vi "ClientNTTestUpdate.vi"(8 "NT Connection":bool, 9 "CreateTestNew":bool, 10 "Flush0":bool, 11 "TestConfig":T1) -> (0 "Value3":dbl, 1 "Value2":dbl, 2 "Value1":dbl, 3 "Value0":dbl, 4 "Good2":bool, 5 "Good1":bool, 6 "Good3":bool, 7 "Good0":bool)   [LabVIEW 2019]
uses:
  ClientNTTestConfig.ctl
  <vilib>/Rock Robotics/Network Tables/NT Read Number.vi
  <vilib>/Rock Robotics/Network Tables/NT Write Number.vi
  <vilib>/Rock Robotics/WPI/ThirdParty/JAS_Junk/TrajLib/Util_GetTime.vi
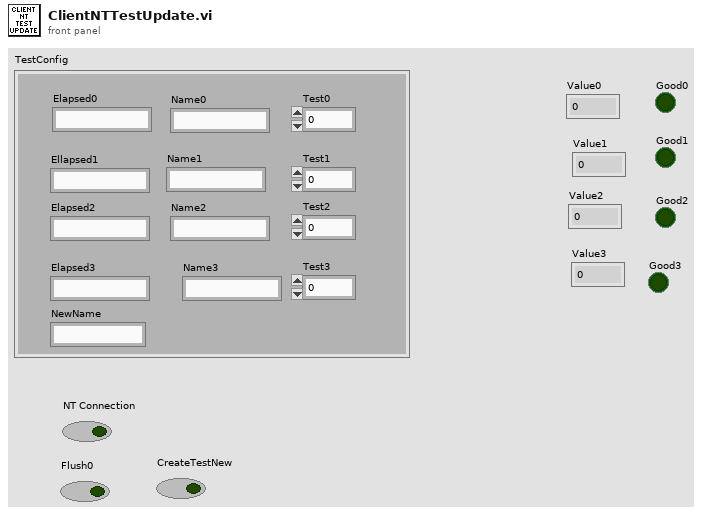
[diagram p1: front panel]
types:
  T1 = typedef "ClientNTTestConfig.ctl" = cluster{"Elapsed0":string, "Name0":string, "Test0":u32, "Ellapsed1":string, "Name1":string, "Test1":u32, "Elapsed2":string, "Name2":string, "Test2":u32, "Elapsed3":string, "Name3":string, "Test3":u32, "NewName":string}
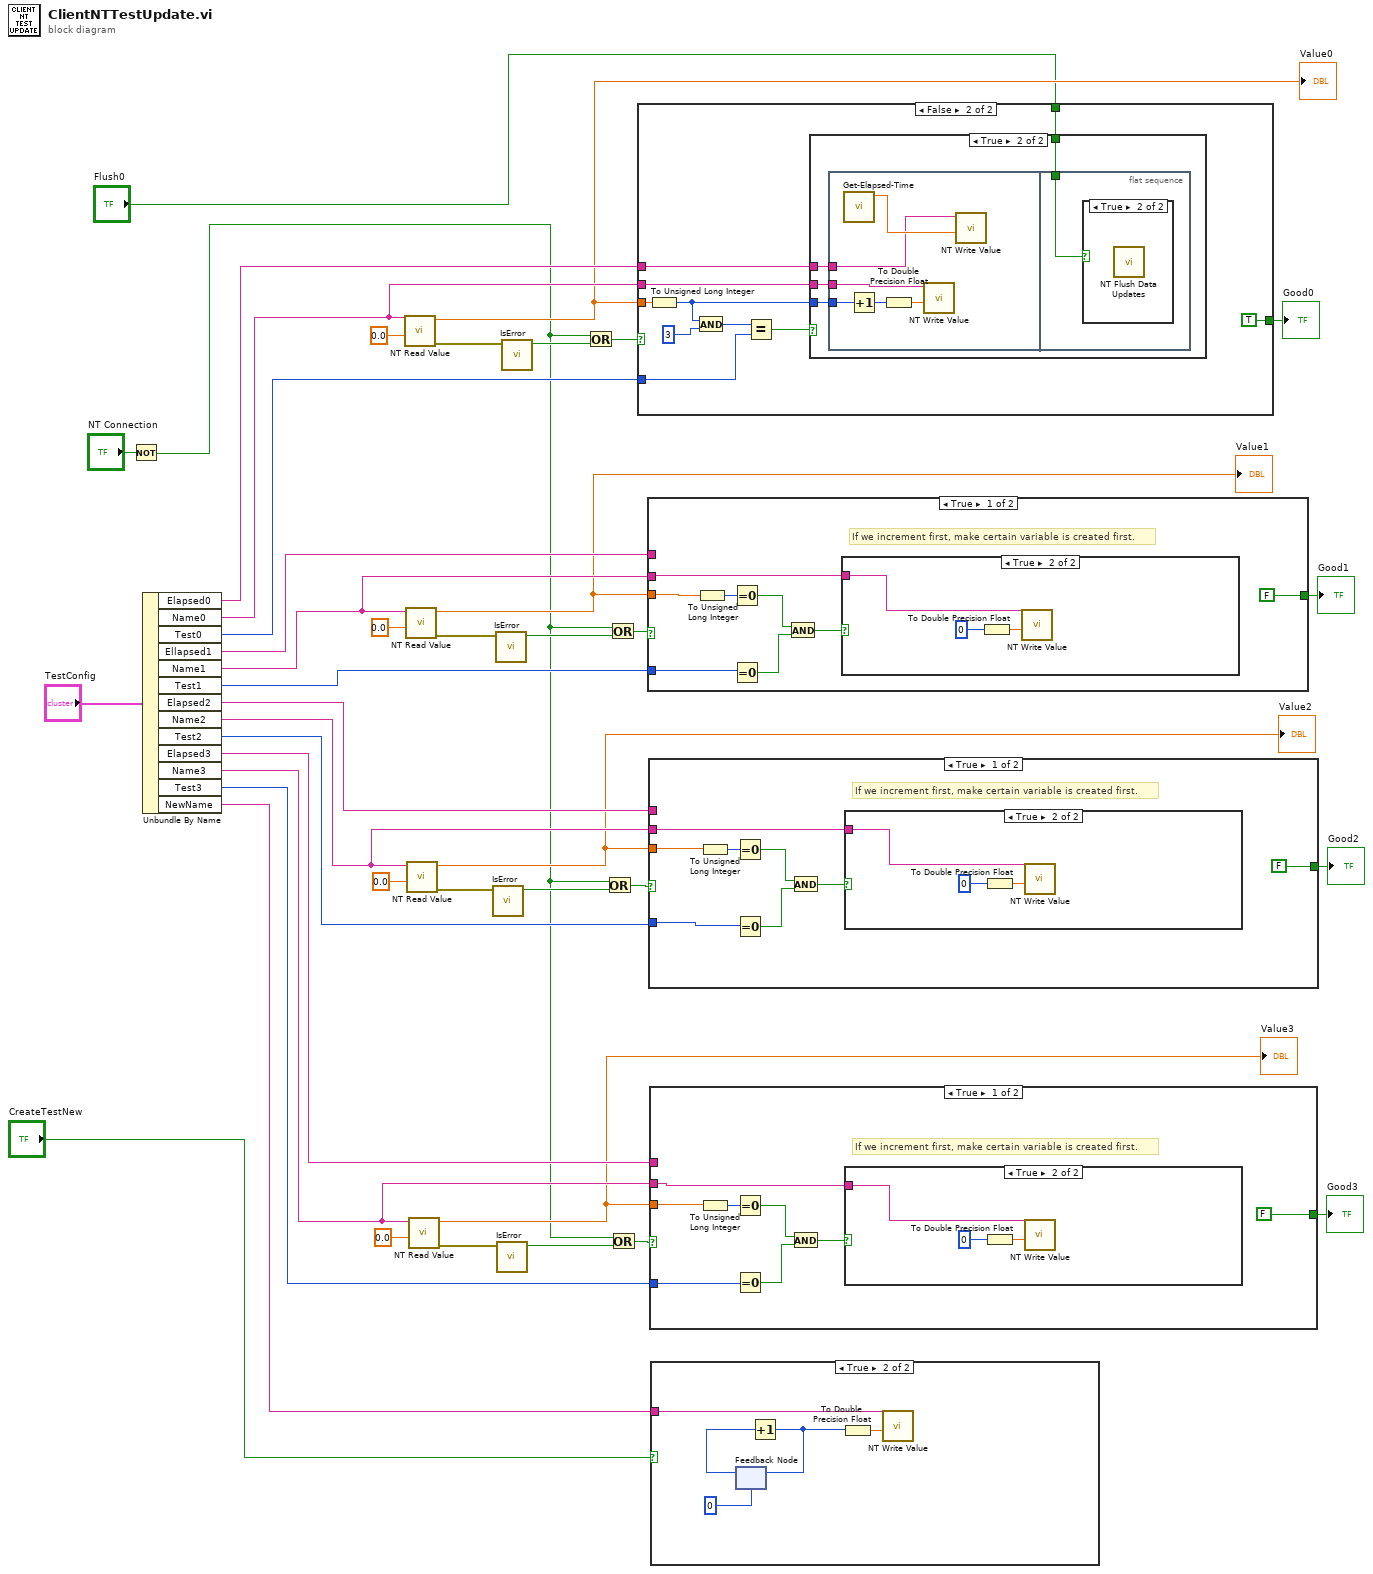
[diagram p0: block diagram]
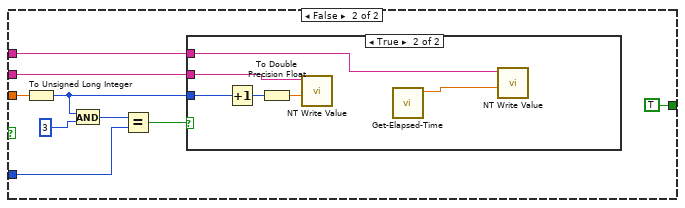
[diagram p4: hidden frame]
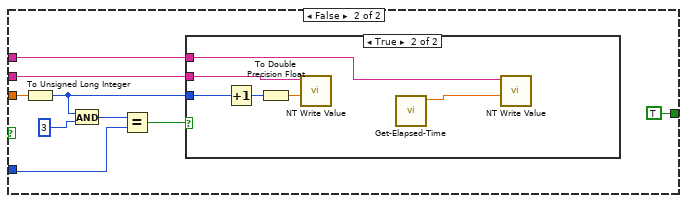
[diagram p7: hidden frame]
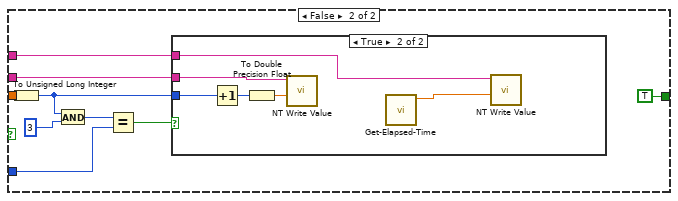
[diagram p10: hidden frame]
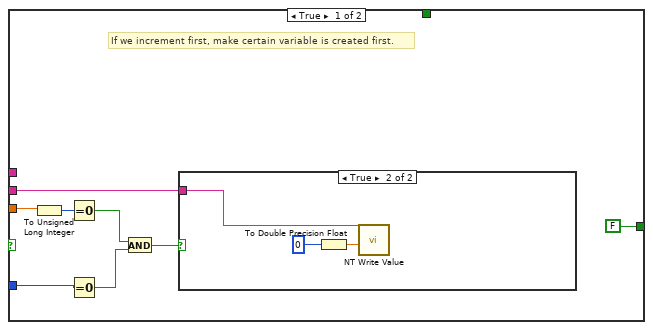
[diagram p12: hidden frame]
diagram:
  n1 = Not(x="NT Connection") -> (.not. x?=w4:bool)
  n2 = Unbundle By Name("TestConfig") -> ("Elapsed0"=w37:string, "Name0"=w36:string, "Test0"=w35:u32, "Ellapsed1"=w34:string, "Name1"=w33:string, "Test1"=w32:u32, "Elapsed2"=w31:string, "Name2"=w30:string, "Test2"=w29:u32, "Elapsed3"=w28:string, "Name3"=w27:string, "Test3"=w26:u32, "NewName"=w2:string)
  n3 = call-poly <vilib>:"NT Read Value.vi"("Default Value"=0.0, "Name"=w36) -> ("error out"=w13:errorcluster, "Numeric"=w22:dbl)  [unwired: 8 in]
  "Value0" <- w22
  n4 = call-poly <vilib>:"NT Read Value.vi"("Default Value"=0.0, "Name"=w33) -> ("error out"=w15:errorcluster, "Numeric"=w25:dbl)  [unwired: 8 in]
  "Value1" <- w25
  n5 = call-poly <vilib>:"NT Read Value.vi"("Default Value"=0.0, "Name"=w30) -> ("error out"=w6:errorcluster, "Numeric"=w24:dbl)  [unwired: 8 in]
  "Value2" <- w24
  n6 = call-poly <vilib>:"NT Read Value.vi"("Default Value"=0.0, "Name"=w27) -> ("error out"=w8:errorcluster, "Numeric"=w23:dbl)  [unwired: 8 in]
  "Value3" <- w23
  n7 = call "IsError.vi"("error in (no error)"=w6) -> ("Boolean"=w10:bool)  [unwired: 10 in]
  n8 = call "IsError.vi"("error in (no error)"=w15) -> ("Boolean"=w14:bool)  [unwired: 10 in]
  n9 = call "IsError.vi"("error in (no error)"=w8) -> ("Boolean"=w9:bool)  [unwired: 10 in]
  n10 = call "IsError.vi"("error in (no error)"=w13) -> ("Boolean"=w12:bool)  [unwired: 10 in]
  n11 = Or(x=w4, y=w12) -> (x .or. y?=w11:bool)
  n12 = Or(x=w4, y=w10) -> (x .or. y?=w5:bool)
  n13 = Or(x=w4, y=w14) -> (x .or. y?=w16:bool)
  n14 = Or(x=w4, y=w9) -> (x .or. y?=w7:bool)
  n15 = case shown="False" w11 {
    tunnel: w37 -> [_ w59]
    tunnel: w36 -> [w44 w58]
    tunnel: w35 -> [w48 w57]
    tunnel: w22 -> [w50 w56]
    tunnel: [FALSE TRUE] -> w21
    tunnel: "Flush0" -> [_ w54]
    frame True {
      # "If we increment first, make certain variable is created first."
      n16 = To Unsigned Long Integer(number=w50) -> (unsigned 32bit integer=w49:u32)
      n17 = Equal To 0?(x=w49) -> (x = 0?=w47:bool)
      n18 = Equal To 0?(x=w48) -> (x = 0?=w46:bool)
      n19 = And(x=w47, y=w46) -> (x .and. y?=w45:bool)
      n20 = case shown="True" w45 {
        tunnel: w44 -> [_ w51]
        frame False {
        }
        frame True {
          n21 = To Double Precision Float(number=u32 0) -> (double precision float=w53:dbl)
          n22 = call-poly <vilib>:"NT Write Value.vi"("Numeric"=w53, "Name"=w51) -> ()  [unwired: 9 in, 1 out]
        }
      }
    }
    frame False {
      n23 = To Unsigned Long Integer(number=w56) -> (unsigned 32bit integer=w62:u32)
      n24 = And(x=w62, y=u32 3) -> (x .and. y?=w63:u32)
      n25 = Equal?(x=w63, y=w57) -> (x = y?=w60:bool)
      n26 = case shown="True" w60 {
        tunnel: w58 -> [_ w66]
        tunnel: w62 -> [_ w67]
        tunnel: w59 -> [_ w65]
        tunnel: w54 -> [_ w64]
        frame False {
        }
        frame True {
          n27 = flat-sequence {
            tunnel: w67 -> [w73]
            tunnel: w66 -> [w72]
            tunnel: w65 -> [w68]
            tunnel: w64 -> [w74]
            frame #0 {
              n28 = call "Get-Elapsed-Time.vi"() -> ("ElapsedTime"=w71:dbl)  [unwired: 11 in]
              n29 = Increment(x=w73) -> (x+1=w70:u32)
              n30 = To Double Precision Float(number=w70) -> (double precision float=w69:dbl)
              n31 = call-poly <vilib>:"NT Write Value.vi"("Numeric"=w69, "Name"=w72) -> ()  [unwired: 9 in, 1 out]
              n32 = call-poly <vilib>:"NT Write Value.vi"("Numeric"=w71, "Name"=w68) -> ()  [unwired: 9 in, 1 out]
            }
            frame #1 {
              n33 = case shown="True" w74 {
                frame False {
                }
                frame True {
                  n34 = call <vilib>:"NT Flush Data Updates.vi"() -> ()  [unwired: 11 in, 1 out]
                }
              }
            }
          }
        }
      }
    }
  }
  "Good0" <- w21
  n35 = case shown="True" w16 {
    tunnel: w34 -> [_ w90]
    tunnel: w33 -> [w78 w89]
    tunnel: w32 -> [w76 w88]
    tunnel: w25 -> [w77 w87]
    tunnel: [FALSE TRUE] -> w20
    frame True {
      # "If we increment first, make certain variable is created first."
      n36 = To Unsigned Long Integer(number=w77) -> (unsigned 32bit integer=w82:u32)
      n37 = Equal To 0?(x=w82) -> (x = 0?=w81:bool)
      n38 = Equal To 0?(x=w76) -> (x = 0?=w80:bool)
      n39 = And(x=w81, y=w80) -> (x .and. y?=w79:bool)
      n40 = case shown="True" w79 {
        tunnel: w78 -> [_ w83]
        frame False {
        }
        frame True {
          n41 = To Double Precision Float(number=u32 0) -> (double precision float=w85:dbl)
          n42 = call-poly <vilib>:"NT Write Value.vi"("Numeric"=w85, "Name"=w83) -> ()  [unwired: 9 in, 1 out]
        }
      }
    }
    frame False {
      n43 = To Unsigned Long Integer(number=w87) -> (unsigned 32bit integer=w93:u32)
      n44 = And(x=w93, y=u32 3) -> (x .and. y?=w94:u32)
      n45 = Equal?(x=w94, y=w88) -> (x = y?=w91:bool)
      n46 = case shown="True" w91 {
        tunnel: w89 -> [_ w99]
        tunnel: w93 -> [_ w100]
        tunnel: w90 -> [_ w95]
        frame False {
        }
        frame True {
          n47 = Increment(x=w100) -> (x+1=w97:u32)
          n48 = To Double Precision Float(number=w97) -> (double precision float=w96:dbl)
          n49 = call-poly <vilib>:"NT Write Value.vi"("Numeric"=w96, "Name"=w99) -> ()  [unwired: 9 in, 1 out]
          n50 = call "Get-Elapsed-Time.vi"() -> ("ElapsedTime"=w98:dbl)  [unwired: 11 in]
          n51 = call-poly <vilib>:"NT Write Value.vi"("Numeric"=w98, "Name"=w95) -> ()  [unwired: 9 in, 1 out]
        }
      }
    }
  }
  "Good1" <- w20
  n52 = case shown="True" w5 {
    tunnel: w31 -> [_ w116]
    tunnel: w30 -> [w102 w115]
    tunnel: w29 -> [w104 w114]
    tunnel: w24 -> [w103 w113]
    tunnel: [FALSE TRUE] -> w19
    frame True {
      # "If we increment first, make certain variable is created first."
      n53 = To Unsigned Long Integer(number=w103) -> (unsigned 32bit integer=w108:u32)
      n54 = Equal To 0?(x=w108) -> (x = 0?=w107:bool)
      n55 = Equal To 0?(x=w104) -> (x = 0?=w106:bool)
      n56 = And(x=w107, y=w106) -> (x .and. y?=w105:bool)
      n57 = case shown="True" w105 {
        tunnel: w102 -> [_ w109]
        frame False {
        }
        frame True {
          n58 = To Double Precision Float(number=u32 0) -> (double precision float=w111:dbl)
          n59 = call-poly <vilib>:"NT Write Value.vi"("Numeric"=w111, "Name"=w109) -> ()  [unwired: 9 in, 1 out]
        }
      }
    }
    frame False {
      n60 = To Unsigned Long Integer(number=w113) -> (unsigned 32bit integer=w119:u32)
      n61 = And(x=w119, y=u32 3) -> (x .and. y?=w120:u32)
      n62 = Equal?(x=w120, y=w114) -> (x = y?=w117:bool)
      n63 = case shown="True" w117 {
        tunnel: w115 -> [_ w125]
        tunnel: w119 -> [_ w126]
        tunnel: w116 -> [_ w121]
        frame False {
        }
        frame True {
          n64 = Increment(x=w126) -> (x+1=w123:u32)
          n65 = To Double Precision Float(number=w123) -> (double precision float=w122:dbl)
          n66 = call-poly <vilib>:"NT Write Value.vi"("Numeric"=w122, "Name"=w125) -> ()  [unwired: 9 in, 1 out]
          n67 = call "Get-Elapsed-Time.vi"() -> ("ElapsedTime"=w124:dbl)  [unwired: 11 in]
          n68 = call-poly <vilib>:"NT Write Value.vi"("Numeric"=w124, "Name"=w121) -> ()  [unwired: 9 in, 1 out]
        }
      }
    }
  }
  "Good2" <- w19
  n69 = case shown="True" w7 {
    tunnel: w28 -> [_ w142]
    tunnel: w27 -> [w130 w141]
    tunnel: w26 -> [w128 w140]
    tunnel: w23 -> [w129 w139]
    tunnel: [FALSE TRUE] -> w18
    frame True {
      # "If we increment first, make certain variable is created first."
      n70 = To Unsigned Long Integer(number=w129) -> (unsigned 32bit integer=w134:u32)
      n71 = Equal To 0?(x=w134) -> (x = 0?=w133:bool)
      n72 = Equal To 0?(x=w128) -> (x = 0?=w132:bool)
      n73 = And(x=w133, y=w132) -> (x .and. y?=w131:bool)
      n74 = case shown="True" w131 {
        tunnel: w130 -> [_ w135]
        frame False {
        }
        frame True {
          n75 = To Double Precision Float(number=u32 0) -> (double precision float=w137:dbl)
          n76 = call-poly <vilib>:"NT Write Value.vi"("Numeric"=w137, "Name"=w135) -> ()  [unwired: 9 in, 1 out]
        }
      }
    }
    frame False {
      n77 = To Unsigned Long Integer(number=w139) -> (unsigned 32bit integer=w145:u32)
      n78 = And(x=w145, y=u32 3) -> (x .and. y?=w146:u32)
      n79 = Equal?(x=w146, y=w140) -> (x = y?=w143:bool)
      n80 = case shown="True" w143 {
        tunnel: w141 -> [_ w151]
        tunnel: w145 -> [_ w152]
        tunnel: w142 -> [_ w147]
        frame False {
        }
        frame True {
          n81 = Increment(x=w152) -> (x+1=w149:u32)
          n82 = To Double Precision Float(number=w149) -> (double precision float=w148:dbl)
          n83 = call-poly <vilib>:"NT Write Value.vi"("Numeric"=w148, "Name"=w151) -> ()  [unwired: 9 in, 1 out]
          n84 = call "Get-Elapsed-Time.vi"() -> ("ElapsedTime"=w150:dbl)  [unwired: 11 in]
          n85 = call-poly <vilib>:"NT Write Value.vi"("Numeric"=w150, "Name"=w147) -> ()  [unwired: 9 in, 1 out]
        }
      }
    }
  }
  "Good3" <- w18
  n86 = case shown="True" "CreateTestNew" {
    tunnel: w2 -> [_ w156]
    frame False {
    }
    frame True {
      n87 = feedback #1(u32 0 ("number")) -> (w154:u32)
      n88 = Increment(x=w154) -> (x+1=w153:u32)
      n89 = feedback-in #1(w153) -> ()
      n90 = To Double Precision Float(number=w153) -> (double precision float=w157:dbl)
      n91 = call-poly <vilib>:"NT Write Value.vi"("Numeric"=w157, "Name"=w156) -> ()  [unwired: 9 in, 1 out]
    }
  }
